vi "core_write_cluster_params_error_handler.vi"(6 "name of caller":string, 8 "error in (no error)":errorcluster, 9 "object name":string, 10 "cluster type":string, 11 "cluster name":string) -> (0 "error out":errorcluster)   [LabVIEW 2015]
uses:
  polys/poly_h5_tools_eco_plus.vi
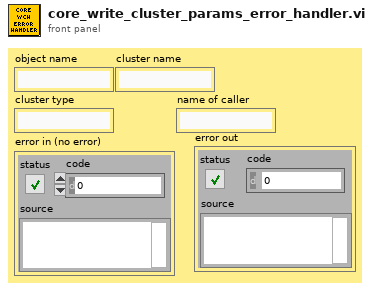
[diagram p1: front panel]
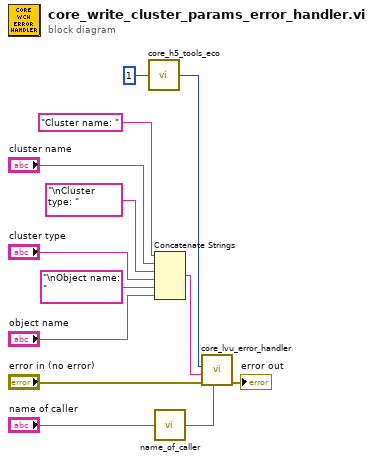
[diagram p0: block diagram]
diagram:
  n1 = call-poly "core_h5_tools_eco.vi"("code (w/out eco)"=1) -> ("code (+ eco)"=w12:i32)  [unwired: 4 in]
  n2 = Concatenate Strings("Cluster name: ", "cluster name", "\nCluster type: ", "cluster type", "\nObject name: ", "object name") -> (w10:string)
  n3 = call "name_of_caller.vi"("name of caller in"="name of caller") -> ("name of caller out"=w9:string)  [unwired: 3 in]
  n4 = call "core_lvu_error_handler.vi"("name of caller in (you)"=w9, "error in (no error)"="error in (no error)", "additional info"=w10, "code (0 = no error)"=w12) -> ("error out"=→"error out":errorcluster)  [unwired: 6 in, 1 out]
